vi "Utility Firmware Version.vi"(5 "Retry Attempts (0)":i32 min=0, 7 "Unit ID (-1)":i32=-1, 9 "error in":errorcluster, 11 "VISA resource name":refnum<visa-resource-name>) -> (1 "error out":errorcluster, 2 "Firmware Version":string, 3 "VISA resource name out":refnum<visa-resource-name>)   [LabVIEW 2020, in "Omega Platinum Series.lvlib"]
doc: "Returns the firmware version string formatted as ##.##.##.## where ## signifies a decimal number."
uses:
  <instrlib>/RxnRover/OmegaPlatinumSeriesDriver/Omega Platinum Series.lvlib
panel:
  out "Command":string
  out "Response":string
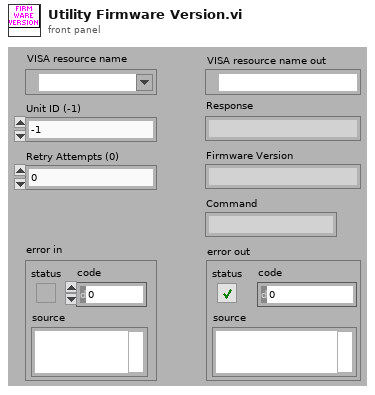
[diagram p1: front panel]
types:
  T1 = typedef "Omega Platinum Series.lvlib/Response.ctl" = cluster{"Unit Address":i32, "Command Class":string, "Command ID":u32, "Parameters":string}
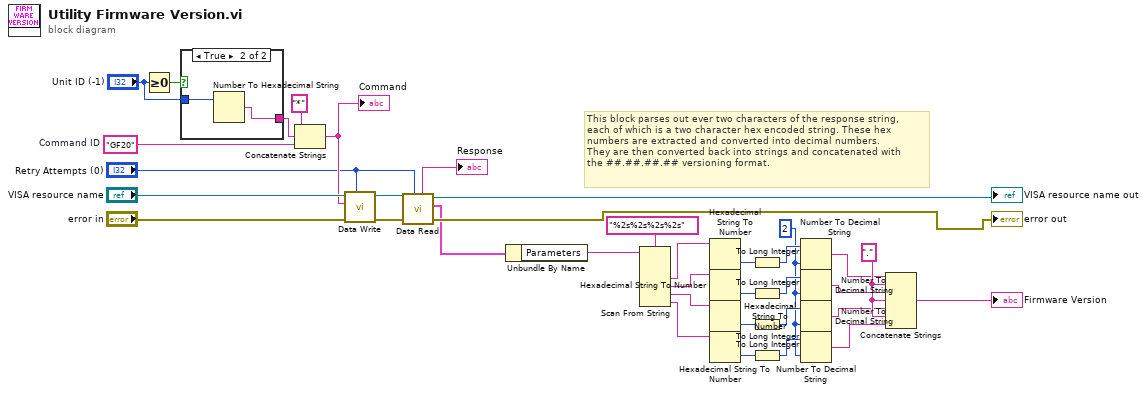
[diagram p0: block diagram]
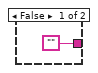
[diagram p2: hidden frame]
diagram:
  w2 = 2
  w30 = "."
  w7 = "GF20"  # Command ID
  # "This block parses out ever two characters of the response string,\neach of which is a two character hex encoded string. These hex\nnumbers are extracted and converted into decimal numbers.\nThey are then converted back into strings and concatenated with\nthe ##.##.##.## versioning format."
  n1 = Greater Or Equal To 0?(x="Unit ID (-1)") -> (x >= 0?=w5:bool)
  n2 = case shown="True" w5 {
    tunnel: "Unit ID (-1)" -> [_ w39]
    tunnel: ["" w38] -> w3
    frame False {
    }
    frame True {
      n3 = Number To Hexadecimal String(2:w39) -> (0:w38:string)  [unwired: 1 in]
    }
  }
  n4 = Concatenate Strings("*" ("string"), w3, w7) -> (w6:string)
  "Command" <- w6
  n5 = call <instrlib>:"Data Write.vi"("Retry Attempts (0)"="Retry Attempts (0)", "error in (no error)"="error in", "Command"=w6, "VISA Refnum in"="VISA resource name") -> ("error out"=w36:errorcluster, "VISA Refnum out"=w35:refnum<visa-resource-name>)  [unwired: 6 in]
  n6 = call <instrlib>:"Data Read.vi"("Retry Attempts (0)"="Retry Attempts (0)", "error in (no error)"=w36, "VISA Refnum in"=w35) -> ("error out"=→"error out":errorcluster, "Response Cluster"=w10:T1, "VISA Refnum out"=→"VISA resource name out":refnum<visa-resource-name>, "read buffer (debug)"=→"Response":string)  [unwired: 5 in]
  n7 = Unbundle By Name(w10) -> ("Parameters"=w32:string)
  n8 = Scan From String(format string="%2s%2s%2s%2s", input string=w32) -> (output 1=w29:string, output 2=w28:string, output 3=w26:string, output 4=w27:string)  [unwired: 6 in, 3 out]
  n9 = Hexadecimal String To Number(string=w29) -> (number=w25:u32)  [unwired: 2 in, 1 out]
  n10 = Hexadecimal String To Number(string=w28) -> (number=w24:u32)  [unwired: 2 in, 1 out]
  n11 = Hexadecimal String To Number(string=w26) -> (number=w23:u32)  [unwired: 2 in, 1 out]
  n12 = Hexadecimal String To Number(string=w27) -> (number=w22:u32)  [unwired: 2 in, 1 out]
  n13 = To Long Integer(number=w25) -> (32bit integer=w21:i32)
  n14 = To Long Integer(number=w24) -> (32bit integer=w20:i32)
  n15 = To Long Integer(number=w23) -> (32bit integer=w19:i32)
  n16 = To Long Integer(number=w22) -> (32bit integer=w18:i32)
  n17 = Number To Decimal String(number=w21, width (-)=w2) -> (decimal integer string=w14:string)
  n18 = Number To Decimal String(number=w20, width (-)=w2) -> (decimal integer string=w17:string)
  n19 = Number To Decimal String(number=w19, width (-)=w2) -> (decimal integer string=w16:string)
  n20 = Number To Decimal String(number=w18, width (-)=w2) -> (decimal integer string=w15:string)
  n21 = Concatenate Strings(w14, w30, w17, w30, w16, w30, w15) -> (→"Firmware Version":string)
